vi "Connect.vi"(8 "error in":errorcluster, 11 "BKPrecision in":refnum<class "9115AT.lvclass">) -> (0 "error out":errorcluster, 3 "BKPrecision out":refnum<class "9115AT.lvclass">)   [LabVIEW 2018, in "9115AT.lvlib" / "9115AT.lvclass"]
uses:
  9115AT.lvclass
  builds/Power_Supply.lvlibp/Power Supply.lvclass
  <instrlib>/BK Precision 911X Series/BK Precision 911X Series.lvlib
  C:/Users/Ron.Dexter.LUMINARTECH/Desktop/builds/Power_Supply.lvlibp/Power Supply.lvclass
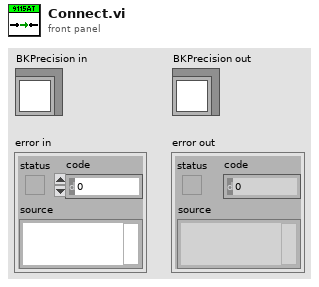
[diagram p1: front panel]
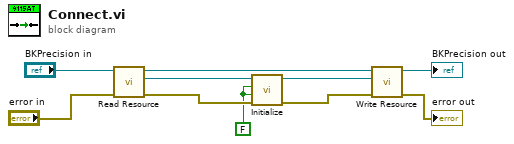
[diagram p0: block diagram]
diagram:
  w1 = FALSE ("ID Query (True)")
  n1 = call "Read Resource.vi"("error in"="error in", "Power Supply in"="BKPrecision in") -> ("error out"=w3:errorcluster, "Resource"=w10:refnum<visa-resource-name>, "Power Supply out"=w8:refnum<class "9115AT.lvclass">)  [unwired: 7 in]
  n2 = call <instrlib>:"Initialize.vi"("error in (no error)"=w3, "Reset (True)"=w1, "ID Query (True)"=w1, "VISA resource name"=w10) -> ("error out"=w2:errorcluster, "VISA resource name out"=w9:refnum<visa-resource-name>)  [unwired: 6 in]
  n3 = call "Write Resource.vi"("error in"=w2, "Resource"=w9, "Power Supply in"=w8) -> ("error out"=→"error out":errorcluster, "Power Supply out"=→"BKPrecision out":refnum<class "9115AT.lvclass">)  [unwired: 7 in]
